vi "Pre-Build Custom Action Generator.vi"() -> (0 "error out":errorcluster)   [LabVIEW 2021]
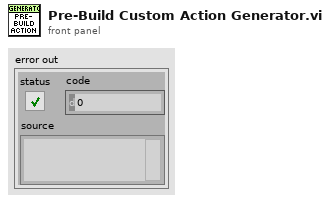
[diagram p1: front panel]
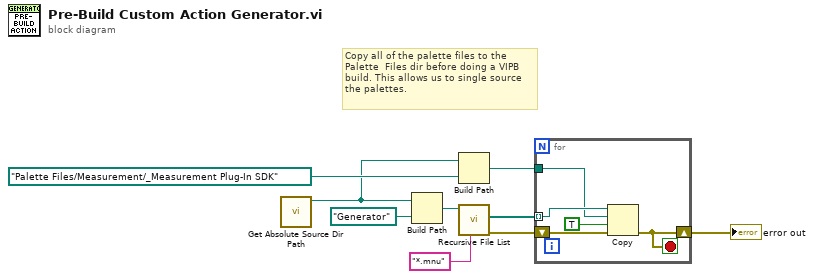
[diagram p0: block diagram]
diagram:
  # "Copy all of the palette files to the \nPalette  Files dir before doing a VIPB\nbuild. This allows us to single source\nthe palettes."
  n1 = call "Get Absolute Source Dir Path.vi"() -> ("source dir"=w2:path)  [unwired: 11 in]
  n2 = Build Path(base path=w2, name or relative path=path "Generator") -> (appended path=w4:path)
  n3 = Build Path(base path=w2, name or relative path=path "Palette Files/Measurement/_Measurement Plug-In SDK") -> (appended path=w3:path)
  n4 = call <vilib>:"Recursive File List.vi"("pattern"="*.mnu", "Folder Path"=w4) -> ("error out"=w7:errorcluster, "All Files in Dir"=w8:path[])  [unwired: 5 in, 3 out]
  n5 = for {
    tunnel: w8 -> [w12] mode=indexing
    tunnel: w3 -> [w11]
    shift-right: [w10] -> w5
    shift-left: w7 -> [w14]
    stop <- w10 stop-if-true
    n6 = Copy(8:w14, 9:TRUE ("overwrite (F)"), 10:w11, 11:w12) -> (0:w10:errorcluster)  [unwired: 1 in, 2 out]
  }
  "error out" <- w5
